vi "AlliGator Update Loaded Dataset Info.vi"(4 "Image Loading Options":T1={"Pixel Well Capacity"=0, "Pile-up Correction"=FALSE, "Gate Step"=0, "Image Smoothing Options"={"Use Image Smoothing"=FALSE, "Kernel Type"=enum."Bilinear", "Bin"=1, "Algorithm"=enum."Rapid"}, "Gates to Skip"={"Start"=0, "End"=0}, "File Background Subtraction"=FALSE, "Background File Path"=path "", "Image Binning Options"={"Use Image Binning"=FALSE, "X Bin"=1, "Y Bin"=1}, "# Gates"=0, "Gates to Keep"={"First"=0, "Last"=0}, "Define Gates to"=FALSE, "Hot Pixel Removal"={"Remove Screamers"=FALSE, "Delta"=0.0, "Equalize Histogram"=FALSE, "Percentile"=0.0, "Hot Pixel Mask Image"=path "", "Use Hot Pixel Mask"=FALSE}, "Dataset Scaling Factor"=0.0, "Image Pre-processing Steps"=[]} {"Hot Pixel Removal"."Percentile" min=0 max=100; "Image Binning Options"."Y Bin" min=1; "Image Binning Options"."X Bin" min=1; "Image Smoothing Options"."Bin" min=1}, 6 "Background File?":bool, 7 "Pile-up Correction":bool, 8 "error in (no error)":errorcluster, 9 "After Loading Dataset Information":T10, 10 "# Gates":i32, 11 "Pixel Well Capacity":u32) -> (0 "Error Out":errorcluster)   [LabVIEW 2021, in "AlliGator Files.lvlib"]
doc: "Updates Settings and Internal Variables after loading a new dataset."
uses:
  AlliGator Files.lvlib
  AlliGator After Loading Dataset Information.ctl
  AlliGator Image Loading Options.ctl
  AlliGator Image Smoothing Options.ctl
  Arrays/Kernel Type.ctl
  Arrays/Smoothing Algorithm.ctl
  AlliGator Gates to Skip.ctl
  AlliGator Image Binning Options.ctl
  AlliGator Gates to Keep.ctl
  SwissSPAD/SwissSPAD Live_Image Display Options.ctl
  AlliGator Image Pre-processing Step.ctl
  AlliGator Variables List.ctl
  AlliGator Settings List.ctl
  AlliGator Refnums List.ctl
  AlliGator Globals, Variables & Constants.lvlib
  AlliGator Settings.lvlib
  AlliGator GUI.lvlib
  Arrays/Arrays.lvlib
  AlliGator Decay Analysis.lvlib
  AlliGator Source Image.lvlib
  SwissSPAD/SwissSPAD Live.lvlib
panel:
  # "see the AlliGator License on the block diagram (Ctrl+E or Window:Show Block Diagram)"
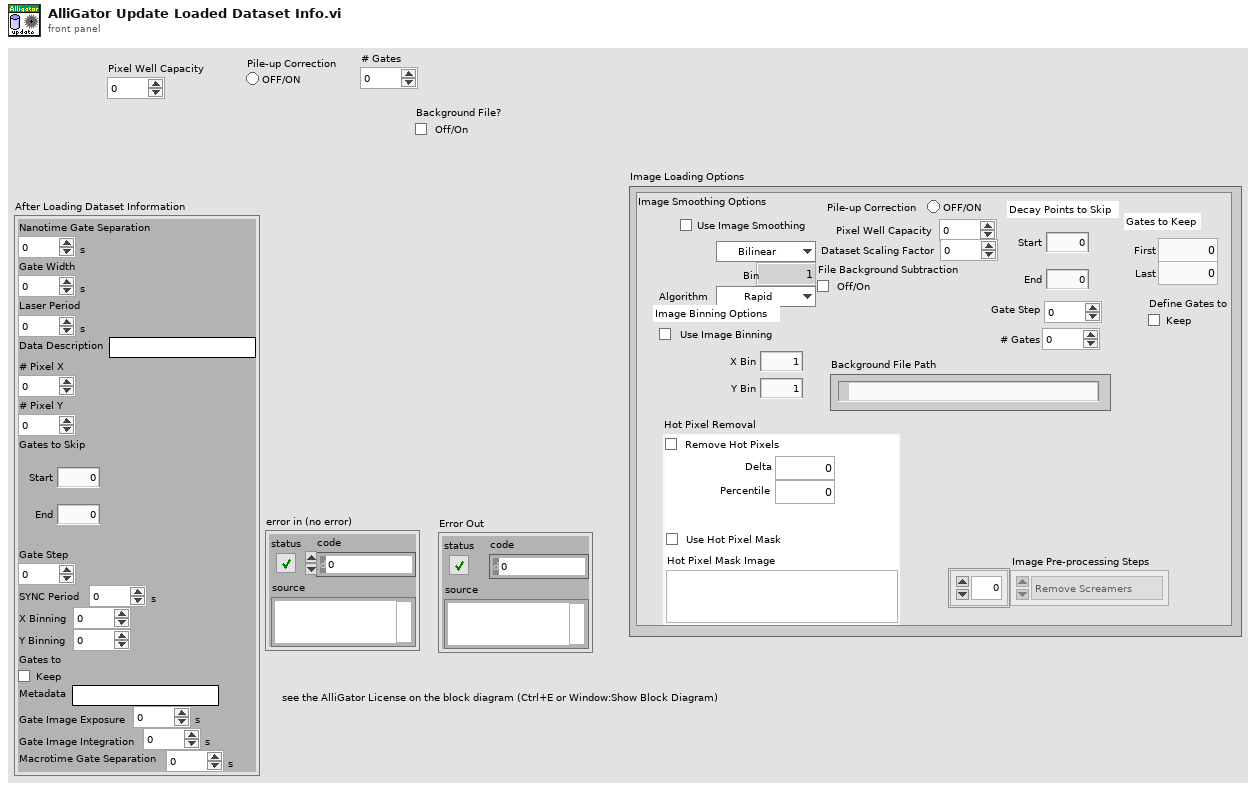
[diagram p1: front panel]
types:
  T1 = typedef "AlliGator Source Image.lvlib/AlliGator Image Loading Options.ctl" = cluster{"Pixel Well Capacity":u32, "Pile-up Correction":bool, "Gate Step":i32, "Image Smoothing Options":T2, "Gates to Skip":T5, "File Background Subtraction":bool, "Background File Path":path, "Image Binning Options":T6, "# Gates":u32, "Gates to Keep":T7, "Define Gates to":bool, "Hot Pixel Removal":T8, "Dataset Scaling Factor":dbl, "Image Pre-processing Steps":T9[]}
  T2 = typedef "AlliGator Settings.lvlib/AlliGator Image Smoothing Options.ctl" = cluster{"Use Image Smoothing":bool, "Kernel Type":T3, "Bin":i32, "Algorithm":T4}
  T3 = typedef "Arrays.lvlib/Kernel Type.ctl" = enum16{"Uniform", "Bilinear", "Gaussian"}
  T4 = typedef "Arrays.lvlib/Smoothing Algorithm.ctl" = enum16{"Rapid", "Thorough"}
  T5 = typedef "AlliGator Decay Analysis.lvlib/AlliGator Gates to Skip.ctl" = cluster{"Start":u32, "End":u32}
  T6 = typedef "AlliGator Source Image.lvlib/AlliGator Image Binning Options.ctl" = cluster{"Use Image Binning":bool, "X Bin":i32, "Y Bin":i32}
  T7 = typedef "AlliGator Settings.lvlib/AlliGator Gates to Keep.ctl" = cluster{"First":u32, "Last":u32}
  T8 = typedef "SwissSPAD Live.lvlib/SwissSPAD Live_Image Display Options.ctl" = cluster{"Remove Screamers":bool, "Delta":sgl, "Equalize Histogram":bool, "Percentile":sgl, "Hot Pixel Mask Image":path, "Use Hot Pixel Mask":bool}
  T9 = typedef "AlliGator Files.lvlib/AlliGator Image Pre-processing Step.ctl" = enum16{"Remove Screamers", "Pile-up Correction", "Binning", "Smoothing", "Rescaling", "Dead Left Column Correction"}
  T10 = typedef "AlliGator Files.lvlib/AlliGator After Loading Dataset Information.ctl" = cluster{"Nanotime Gate Separation":dbl[unit], "Gate Width":dbl[unit], "Laser Period":dbl[unit], "Data Description":string, "# Pixel X":i32, "# Pixel Y":i32, "Gates to Use":cluster{"Start":u32, "End":u32}, "Gate Step":i32, "SYNC Period":dbl[unit], "X Binning":i32, "Y Binning":i32, "Gates to":bool, "Metadata":string, "Gate Image Exposure":dbl[unit], "Gate Image Integration":dbl[unit], "Macrotime Gate Separation":dbl[unit]}
  T11 = typedef "AlliGator Globals, Variables & Constants.lvlib/AlliGator Variables List.ctl" = enum16{"---- GUI ----", "Initialization Status", "State Indicators Refnum", "Original AlliGator Menu Items", "Current Action Loop State", "Script in progress", "Playback", "Loop Playback", "Search ROI Used", "Search ROI", "Decay Graph Max Legend Size", "Intensity Graph Max Legend Size", "Decay Statistics Graph Max Legend Size", "Phasor Graph Max Legend Size", "Phasor Ratio Graph Max Legend Size", "Lifetime Graph Max Legend Size", "---- Files ----", "Export Dataset Frames as Individual Files", "Show Batch Export Help Balloons", "Frames in Dataset", "ptu File Frame Start Indices", "Current Frame in Dataset", "Current Frame Timestamp", "------ Python Plugins ------", "Python Plugins Information", "Python Session", "Valid Python Session?", "---- Source Image ----", "Dataset Loaded", "Dataset Metadata", "Dataset Channel", "Dataset Data Description", "Background Dataset Metadata", "Background Dataset Channel", "Background Dataset Data Description", "Background File Subtraction", "Background File Path", "Background File Pile-up Correction", "Background File Pixel Well Capacity", "Background File Scaling Factor", "Source Image ROIs", "Current Source Image ROI", "Source Image ROI Event Refnum", "X_Source Image Display Range", "X_Source Image Palette Information", "Source Image Palette List", "Source Image Scale", "Current Dataset Load Settings", "Source Image:ROI Overlay Color", "---- Image Profile Window ----", "Image Profile:Overlay ROI in Source Image", "Image Profile Window Event Refnum", "Image Profile:IntensityType", "Image Profile:Intensity Average Type", "Image Profile:Intensity-weighted SDV", "Image Profile:Box Profile Type", "Image Profile Window Open", "Image Profile:Plotted Fit Parameter", "X_Type of Displayed Image", "X_Time Gate Slider", "Dataset Path", "Source Image Overlay to Erase", "Is Displayed Image Accumulated", "White Light Image Modified", "Mask Image Modified", "Macrotime Gate Separation", "------ Phasor Graph -------", "Phasor Graph:Show Line", "---- Phasor Plot ---", "Phasor Plot Parameters Changed", "FLI Dataset Modified since last Phasor Plot Calculation", "Phasor Harmonics Data", "Selected Phasor Harmonics", "Phasor Harmonic Manager Event Refnum", "Phasor Plot ROIs", "Current Phasor Plot ROI", "Phasor Plot ROI Event Refnum", "Phasor Plot Image Reference Points", "Phasor Plot Computed", "Phasor Plot Palette Information", "Phasor Plot Palette List", "Phasor Ratio Palette Information", "Phasor Ratio Palette List", "Phasor Image Scale", "Phasor Plot Image Overlay to Erase", "Phasor Plot Image Elements to Update", "Current Phasor Plot Calculation Parameters", "Current Phasor Calibration Options", "Reset Cumulated Phasor Plot", "Phasor Ratio Reference 1", "Phasor Ratio Lifetime Reference 1", "Phasor Ratio Reference 1 Frequency", "Phasor Ratio Reference 2", "Phasor Ratio Lifetime Reference 2", "Phasor Ratio Reference 2 Frequency", "---- Decay Analysis ----", "Number of Selected Decays to Fit", "LS Fit Results", "LAR Fit Results", "BS Fit Results", "Last Decay Max - Min", "Best Fit Parameters", "Best Fit Parameter Names", "Actual Size X", "Actual Size Y", "Binning X", "Binning Y", "Actual # Gates", "Dataset Number", "Gates to...", "Gates Skipped", "Gates to keep", "Gate Step", "Gate Separation", "Reversed Gates", "Pile-up Correction", "Pixel Well Capacity", "Background Subtracted", "Background Subtraction Method", "Background Definition Range", "Background File (deprecated)", "Number of Dataset Accumulated", "Array of Accumulated Dataset Paths", "Do Averaged Datasets", "Destination File Path", "Process Plot Target", "Use 1/D as Phasor Frequency", "---- Decay Fit Parameter Map -----", "Decay Fit Parameter Map Palette Information", "Decay Fit Parameter Map Palette List", "Local Decay Graph Window Event Refnum", "------- Local Decay Window ---------", "Use normalized IRF for convolution", "----- Miscellaneous ----", "Skippable Dialog Windows Status"}
  T12 = typedef "AlliGator Settings.lvlib/AlliGator Settings List.ctl" = enum16{"GUI:Visible Settings Tab", "GUI:Last Run Version", "Source Image:Use Image Histogram for Contrast", "Source Image:Low Count Pixels Rejection Options", "Source Image:High Count Pixels Rejection Options", "Source Image:Use Image Brightness", "Source Image:Blend Overlay with Image Background", "Source Image:Use Fixed ROI Diameter", "Source Image:ROI Diameter", "Source Image:ROI Center Color", "Source Image:Peak Threshold", "Source Image:Intensity Threshold", "Source Image:Image Binning Options", "Source Image:Image Smoothing Options", "Source Image:Image Histogram Active", "Source Image:Invert Binary Mask", "Source Image:Hot Pixel Removal", "Source Image:Overlay Analyzed ROI Center", "Source Image:Auto-Adjust Contrast", "Source Image:Histogram Lower Percentile", "Source Image:Histogram Upper Percentile", "Source Image:Save Source Image", "Source Image:Scale Bar Options", "Source Image:Image Resolution (Pixel Size)", "Source Image:Flatfield Correction", "Source Image:Show Dead Left Columns Correction", "Source Image:Dead Left Columns Correction", "Source Image:Image Pre-Processing Operations Order", "Data Information:Gate Width", "Data Information:Nanotime Gate Separation", "Data Information:Macrotime Gate Separation", "Data Information:Gate Step", "Data Information:# Gates", "Data Information:Gate Image Exposure", "Data Information:Gate Image Integration", "Data Information:Gates to Skip", "Data Information:Gates to Keep", "Data Information:Define Gates to", "Data Information:Channel Name", "Data Information:Available Channel Names", "Data Information:Channel Arithmetic", "Data Information:Background File Subtraction", "Data Information:Background File", "Data Information:Background Scaling Factor", "Data Information:Background Pile-up Correction", "Data Information:Background Pixel Well Capacity", "Data Information:Laser Period", "Data Information:SYNC Period", "Data Information:Pile-up Correction", "Data Information:Pixel Well Capacity", "Data Information:Dataset Scaling Factor", "Fluorescence Decay_Decay Pre-Processing:Reverse Gates", "Fluorescence Decay_Decay Pre-Processing:Verbose Decay Pre-Processing", "Fluorescence Decay_Decay Pre-Processing:Use Decay Pre-Processing", "Fluorescence Decay_Decay Pre-Processing:Background Subtraction", "Fluorescence Decay_Decay Pre-Processing:Background Definition Range", "Fluorescence Decay_Decay Pre-Processing:Baseline Subtraction Method", "Fluorescence Decay_Decay Pre-Processing:Decay Pre-Processing Operations Order", "Fluorescence Decay_Decay Pre-Processing:Smoothing Parameter", "Fluorescence Decay_Decay Pre-Processing:Shift Decay", "Fluorescence Decay_Decay Pre-Processing:Decay Shift Parameters", "Fluorescence Decay_Decay Pre-Processing:Fold Decay", "Fluorescence Decay_Decay Pre-Processing:# Folds", "Fluorescence Decay_Decay Pre-Processing:1-Normalize Decay", "Fluorescence Decay_Decay Pre-Processing:[0-1]-Normalize Decay", "Fluorescence Decay_Decay Pre-Processing:Smoothen Decay", "Fluorescence Decay_Decay Pre-Processing:Extrapolate Decay", "Fluorescence Decay_Decay Pre-Processing:Use Periodicity", "Fluorescence Decay_Decay Pre-Processing:Use Cursors", "Fluorescence Decay_Decay Pre-Processing:Tail Fraction", "Fluorescence Decay_Decay Pre-Processing:Head Fraction", "Fluorescence Decay_Decay Pre-Processing:Additional Points", "Fluorescence Decay_Decay Pre-Processing:Straighten Decay", "Fluorescence Decay_Decay Pre-Processing:Constant Background", "Fluorescence Decay_Decay Pre-Processing:Pixel-Normalize Decay", "Fluorescence Decay_Advanced Analysis:Extract IRF instead of Decay", "Fluorescence Decay_Advanced Analysis:IRF Extraction Options", "Fluorescence Decay_Advanced Analysis:IRF Optimization Options", "Fluorescence Decay_Advanced Analysis:Square Pulse Options", "Fluorescence Decay_Advanced Analysis:IRF Order", "Fluorescence Decay_Advanced Analysis:IRF Time Constants", "Fluorescence Decay_Advanced Analysis:Wavelet Analysis Options", "Fluorescence Decay_Advanced Analysis:Average Lifetime Options", "Fluorescence Decay_Fit Options:Fit Options", "Fluorescence Decay_Fit Options:Use Legacy Fitting Approach", "Fluorescence Decay_Fit Options:Use Data Information Laser Period", "Fluorescence Decay_Fit Parameters:Displayed Fit Parameters", "Fluorescence Decay_Fit Parameters:Fit Parameter Constraints", "Fluorescence Decay_Fit Parameters:Export Tabulated Results", "Fluorescence Decay_Fit Parameters:MLE Baseline Offset Type", "Fluorescence Decay_Fit Parameters:MLE Baseline Offset", "Fluorescence Decay_Fit Parameters:Guess Parameter Names", "Fluorescence Decay_Fit Parameters:Guess Parameter Values", "Fluorescence Decay_Fit Parameters:Guess Parameters Options", "Fluorescence Decay_Styles:Show Last Decay Only", "Fluorescence Decay_Styles:Decay Graph Color Array", "Fluorescence Decay:Decay Graph Active", "Fluorescence Decay Statistics:Min Peak Value", "Fluorescence Decay Statistics:Reject Low Decay Peak Pixels", "Fluorescence Decay Statistics:Reject High Decay Peak Pixels", "Fluorescence Decay Statistics:Max Peak Value", "Time Traces:Use File Timestamp", "Time Traces:Time Step", "Time Traces:Use Intensity Correction File", "Time Traces:Intensity Correction File", "Phasor Plot:Phasor Plot Smoothing Options", "Phasor Plot:Phasor Plot Size", "Phasor Plot:Phasor Plot Graphics Options", "Phasor Plot:Cumulative Phasor Plot", "Phasor Plot:Use Phasor Brightness", "Phasor Plot:Blend Overlay with Phasor Background", "Phasor Plot:Save Phasor Plot", "Phasor Plot:Show References", "Phasor Plot:Phasor Ratio Decay Range", "Phasor Plot:Exponential Fading", "Phasor Plot:Phasor Ratio Reference Colors", "Phasor Plot:Reference Radius", "Phasor Plot:Show Color Map Vertices", "Phasor Plot:Phasor Plot Active", "Phasor Plot:Phasor Ratio Color Map Type", "Phasor Plot:Phasor Ratio Color Map", "Phasor Plot:Phasor Ratio Display Range", "Phasor Plot:Selected Image ROI(s)", "Phasor Plot:All Image ROIs", "Phasor Plot:Selected Phasor Plot ROI(s)", "Phasor Plot:All Phasor Plot ROIs", "Phasor Plot:Phasor Ratio Color-Coded Quantity", "Phasor Plot:Store Phasor Harmonics", "Phasor Plot:Draw Reference Segment", "Phasor Plot:User-Defined Quantity", "Phasor Graph:Phasor Frequency", "Phasor Graph:Phasor Ratio Type", "Phasor Graph:Pixel-level Phasor Computation", "Phasor Graph:Save Phasor Graph", "Phasor Graph:Phasor Graph Active", "Phasor Graph:Phasor SDV Options", "Phasor Calibration:Use Backup Calibration if needed", "Phasor Graph:Define Shortest Lifetime as", "Phasor Calibration:Backup Calibration Type", "Phasor Calibration:Calibration Type", "Phasor Calibration:Calibration Lifetime", "Phasor Calibration:Calibration Map Algorithm", "Single-Exponential Phasor Locus (SEPL):Gate Parameters", "Single-Exponential Phasor Locus (SEPL):User-defined Gate", "Single-Exponential Phasor Locus (SEPL):User-defined IRF", "Single-Exponential Phasor Locus (SEPL):Phasor Parameters", "Single-Exponential Phasor Locus (SEPL):Decay & IRF Parameters", "Single-Exponential Phasor Locus (SEPL):Display Parameters", "Lifetime Analysis:Decay Analysis Parameters", "Lifetime Analysis:Lifetime Map Active", "Plugins:Python Settings", "Miscellaneous:Verbose Mode", "Miscellaneous:Beep after Script", "Miscellaneous:Saved Image File Format", "Miscellaneous:Exported Gate Image Settings", "Miscellaneous:Include Loading in Timing", "Miscellaneous:Verbose Settings Mode", "Miscellaneous:Histogram Options", "Miscellaneous:Beep on Error", "Miscellaneous:# Logical Processors Used", "Miscellaneous:ROI Description Max Characters", "Miscellaneous:Verbose Error Mode", "Miscellaneous:Transparent Mask Color"}
  T13 = typedef "AlliGator Globals, Variables & Constants.lvlib/AlliGator Refnums List.ctl" = enum16{"---------- AlliGator Controls ----------", "AlliGator Tab Control Refnum", "---------- AlliGator Indicators ----------", "Source Image Display Refnum", "Phasor Plot Display Refnum", "Decay Fit Parameter Map Refnum", "---------- AlliGator VIs ----------", "AlliGator Settings Refnum", "AlliGator Launcher Refnum"}
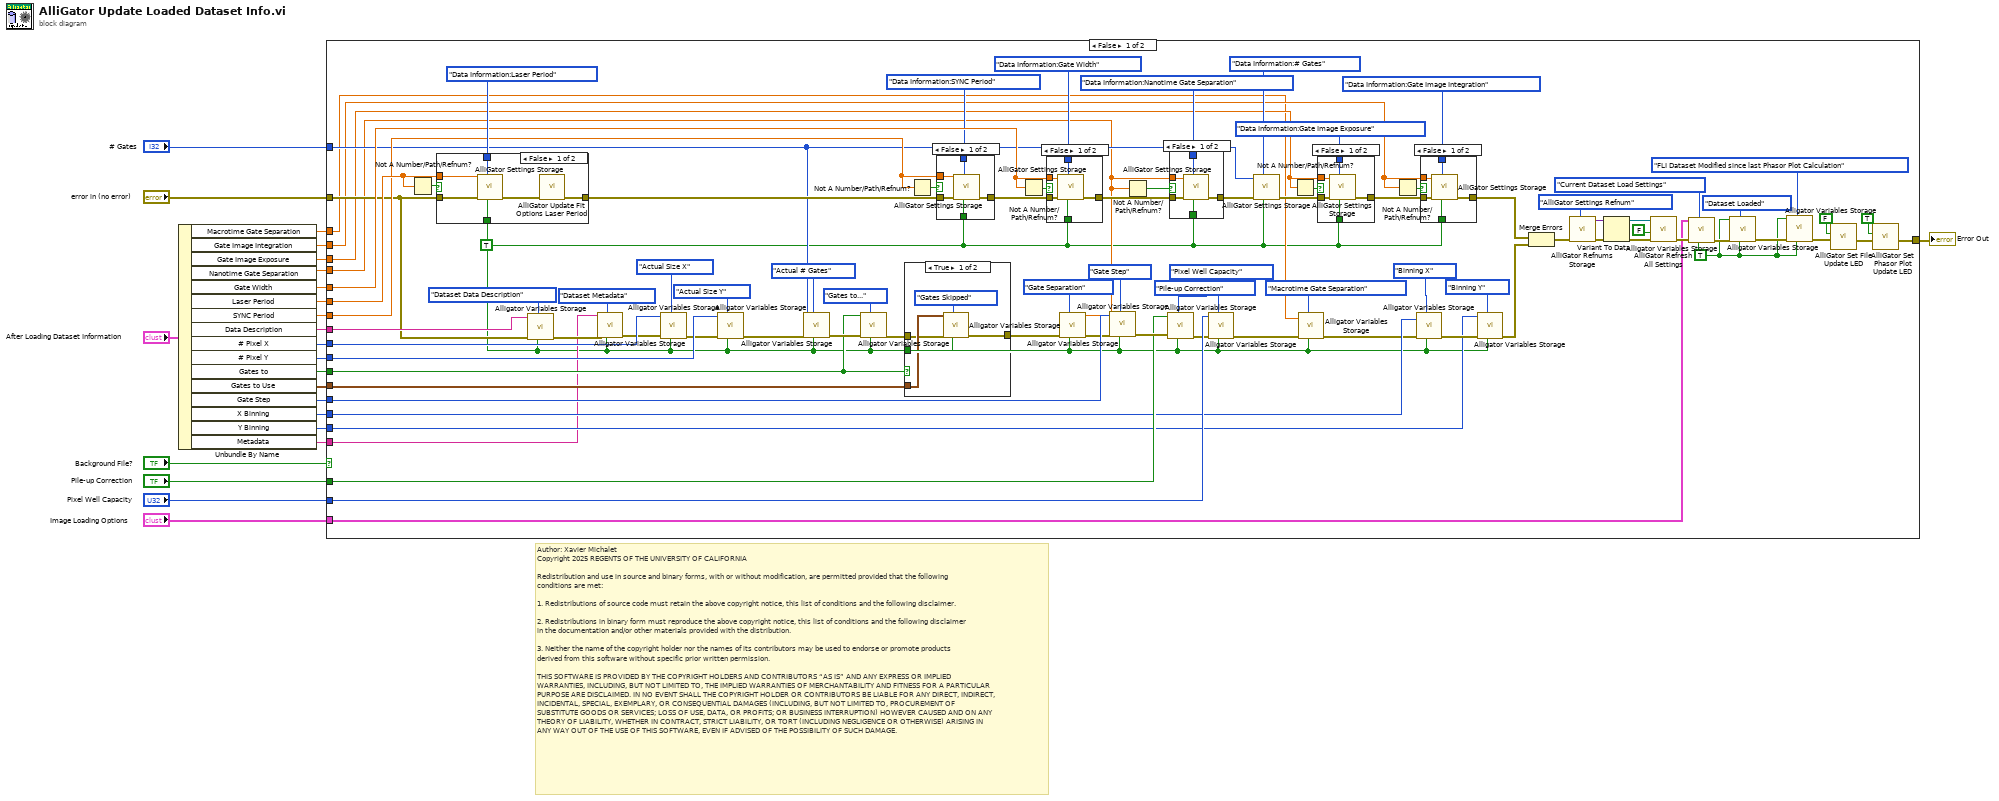
[diagram p0: block diagram]
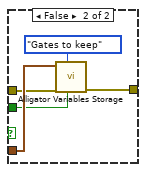
[diagram p6: hidden frame]
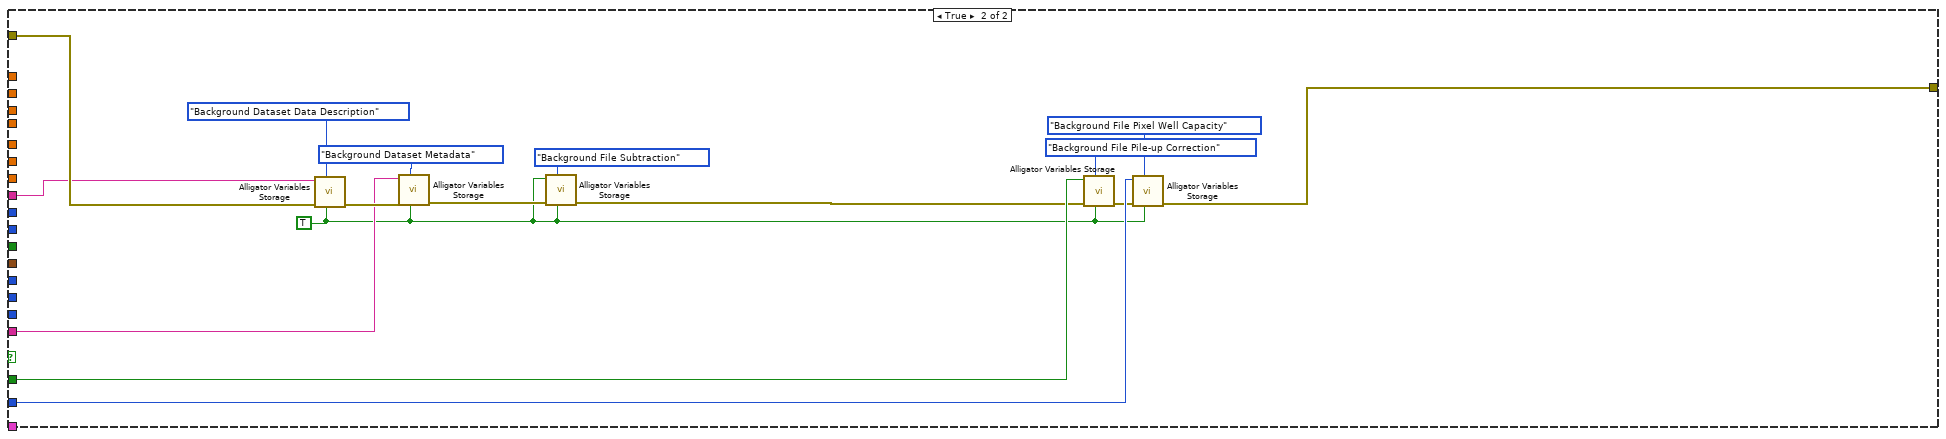
[diagram p9: hidden frame]
diagram:
  # "Author: Xavier Michalet\nCopyright 2025 REGENTS OF THE UNIVERSITY OF CALIFORNIA\n\nRedistribution and use in source and binary forms, with or without modification, are permitted provided that the following conditions are met:\n\n1. Redistributions of source code must retain the above copyright notice, this list of conditions and the following disclaimer.\n\n2. Redistributions in binary form must reproduce the above copyright notice, this list of conditions and the following disclaimer in the documentation and/or other materials provided with the distribution.\n\n3. Neither the name of the copyright holder nor the names of its contributors may be used to endorse or promote products derived from this software without specific prior written permission.\n\nTHIS SOFTWARE IS PROVIDED BY THE COPYRIGHT HOLDERS AND CONTRIBUTORS “AS IS” AND ANY EXPRESS OR IMPLIED WARRANTIES, INCLUDING, BUT NOT LIMITED TO, THE IMPLIED WARRANTIES OF MERCHANTABILITY AND FITNESS FOR A PARTICULAR PURPOSE ARE DISCLAIMED. IN NO EVENT SHALL THE COPYRIGHT HOLDER OR CONTRIBUTORS BE LIABLE FOR ANY DIRECT, INDIRECT, INCIDENTAL, SPECIAL, EXEMPLARY, OR CONSEQUENTIAL DAMAGES (INCLUDING, BUT NOT LIMITED TO, PROCUREMENT OF SUBSTITUTE GOODS OR SERVICES; LOSS OF USE, DATA, OR PROFITS; OR BUSINESS INTERRUPTION) HOWEVER CAUSED AND ON ANY THEORY OF LIABILITY, WHETHER IN CONTRACT, STRICT LIABILITY, OR TORT (INCLUDING NEGLIGENCE OR OTHERWISE) ARISING IN ANY WAY OUT OF THE USE OF THIS SOFTWARE, EVEN IF ADVISED OF THE POSSIBILITY OF SUCH DAMAGE."
  n1 = Unbundle By Name("After Loading Dataset Information") -> ("Macrotime Gate Separation"=w1:dbl[unit], "Gate Image Integration"=w2:dbl[unit], "Gate Image Exposure"=w3:dbl[unit], "Nanotime Gate Separation"=w8:dbl[unit], "Gate Width"=w17:dbl[unit], "Laser Period"=w18:dbl[unit], "SYNC Period"=w15:dbl[unit], "Data Description"=w10:string, "# Pixel X"=w22:i32, "# Pixel Y"=w23:i32, "Gates to"=w11:bool, "Gates to Use"=w24:cluster{"Start":u32, "End":u32}, "Gate Step"=w14:i32, "X Binning"=w13:i32, "Y Binning"=w12:i32, "Metadata"=w4:string)
  n2 = case shown="False" "Background File?" {
    tunnel: w24 -> [w112 _]
    tunnel: w23 -> [w111 _]
    tunnel: w22 -> [w110 _]
    tunnel: "Pile-up Correction" -> [w106 w175]
    tunnel: "Pixel Well Capacity" -> [w105 w174]
    tunnel: w18 -> [w95 _]
    tunnel: w17 -> [w93 _]
    tunnel: "# Gates" -> [w40 _]
    tunnel: w15 -> [w85 _]
    tunnel: w14 -> [w81 _]
    tunnel: w13 -> [w76 _]
    tunnel: w12 -> [w75 _]
    tunnel: w11 -> [w64 _]
    tunnel: w10 -> [w63 w167]
    tunnel: "error in (no error)" -> [w61 w168]
    tunnel: w8 -> [w31 _]
    tunnel: [w53 w173] -> w6
    tunnel: "Image Loading Options" -> [w48 _]
    tunnel: w4 -> [w44 w169]
    tunnel: w3 -> [w33 _]
    tunnel: w2 -> [w32 _]
    tunnel: w1 -> [w27 _]
    frame False {
      w49 = TRUE ("Get(F)/Set")
      w25 = TRUE ("Get(F)/Set")
      n3 = Not A Number/Path/Refnum?(number/path/refnum=w95) -> (NaN/Path/Refnum?=w94:bool)
      n4 = case shown="False" w94 {
        tunnel: w25 -> [w158 _]
        tunnel: [w154 w159] -> w88
        tunnel: AlliGator_Settings_List."Data Information:Laser Period" ("AlliGator Settings List") -> [w157 _]
        tunnel: w95 -> [w153 _]
        tunnel: w61 -> [w156 w159]
        frame False {
          n5 = call "AlliGator Settings Storage.vi"("Get(F)/Set"=w158, "AlliGator Settings List"=w157, "Error In"=w156, "Variant Data in"=w153) -> ("Error Out"=w155:errorcluster)  [unwired: 6 in, 1 out]
          n6 = call "AlliGator Update Fit Options Laser Period.vi"("error in (no error)"=w155) -> ("error out"=w154:errorcluster)  [unwired: 10 in]
        }
        frame True {
        }
      }
      n7 = call "Alligator Variables Storage.vi"("Get(F)/Set"=w25, "AlliGator Variable"=AlliGator_Variables_List."Dataset Data Description" ("Alligator Variable"), "Error In"=w61, "Data in"=w63) -> ("Error Out"=w47:errorcluster)  [unwired: 5 in, 2 out]
      n8 = call "Alligator Variables Storage.vi"("Get(F)/Set"=w25, "AlliGator Variable"=AlliGator_Variables_List."Dataset Metadata" ("Alligator Variable"), "Error In"=w47, "Data in"=w44) -> ("Error Out"=w46:errorcluster)  [unwired: 5 in, 2 out]
      n9 = call "Alligator Variables Storage.vi"("Get(F)/Set"=w25, "AlliGator Variable"=AlliGator_Variables_List."Actual Size X" ("Alligator Variable"), "Error In"=w46, "Data in"=w110) -> ("Error Out"=w101:errorcluster)  [unwired: 5 in, 2 out]
      n10 = call "Alligator Variables Storage.vi"("Get(F)/Set"=w25, "AlliGator Variable"=AlliGator_Variables_List."Actual Size Y" ("Alligator Variable"), "Error In"=w101, "Data in"=w111) -> ("Error Out"=w103:errorcluster)  [unwired: 5 in, 2 out]
      n11 = call "Alligator Variables Storage.vi"("Get(F)/Set"=w25, "AlliGator Variable"=AlliGator_Variables_List."Actual # Gates" ("Alligator Variable"), "Error In"=w103, "Data in"=w40) -> ("Error Out"=w67:errorcluster)  [unwired: 5 in, 2 out]
      n12 = call "Alligator Variables Storage.vi"("Get(F)/Set"=w25, "AlliGator Variable"=AlliGator_Variables_List."Gates to..." ("Alligator Variable"), "Error In"=w67, "Data in"=w64) -> ("Error Out"=w66:errorcluster)  [unwired: 5 in, 2 out]
      n13 = case shown="True" w64 {
        tunnel: w112 -> [w141 w146]
        tunnel: [w139 w144] -> w83
        tunnel: w66 -> [w138 w143]
        tunnel: w25 -> [w137 w142]
        frame True {
          n14 = call "Alligator Variables Storage.vi"("Get(F)/Set"=w137, "AlliGator Variable"=AlliGator_Variables_List."Gates Skipped" ("Alligator Variable"), "Error In"=w138, "Data in"=w141) -> ("Error Out"=w139:errorcluster)  [unwired: 5 in, 2 out]
        }
        frame False {
          n15 = call "Alligator Variables Storage.vi"("Get(F)/Set"=w142, "AlliGator Variable"=AlliGator_Variables_List."Gates to keep" ("Alligator Variable"), "Error In"=w143, "Data in"=w146) -> ("Error Out"=w144:errorcluster)  [unwired: 5 in, 2 out]
        }
      }
      n16 = Not A Number/Path/Refnum?(number/path/refnum=w85) -> (NaN/Path/Refnum?=w86:bool)
      n17 = case shown="False" w86 {
        tunnel: w25 -> [w151 _]
        tunnel: [w150 w152] -> w87
        tunnel: AlliGator_Settings_List."Data Information:SYNC Period" ("AlliGator Settings List") -> [w149 _]
        tunnel: w85 -> [w148 _]
        tunnel: w88 -> [w147 w152]
        frame False {
          n18 = call "AlliGator Settings Storage.vi"("Get(F)/Set"=w151, "AlliGator Settings List"=w149, "Error In"=w147, "Variant Data in"=w148) -> ("Error Out"=w150:errorcluster)  [unwired: 6 in, 1 out]
        }
        frame True {
        }
      }
      n19 = Not A Number/Path/Refnum?(number/path/refnum=w93) -> (NaN/Path/Refnum?=w92:bool)
      n20 = case shown="False" w92 {
        tunnel: w25 -> [w135 _]
        tunnel: [w134 w136] -> w107
        tunnel: AlliGator_Settings_List."Data Information:Gate Width" ("AlliGator Settings List") -> [w133 _]
        tunnel: w87 -> [w132 w136]
        tunnel: w93 -> [w131 _]
        frame False {
          n21 = call "AlliGator Settings Storage.vi"("Get(F)/Set"=w135, "AlliGator Settings List"=w133, "Error In"=w132, "Variant Data in"=w131) -> ("Error Out"=w134:errorcluster)  [unwired: 6 in, 1 out]
        }
        frame True {
        }
      }
      n22 = call "Alligator Variables Storage.vi"("Get(F)/Set"=w25, "AlliGator Variable"=AlliGator_Variables_List."Gate Separation" ("Alligator Variable"), "Error In"=w83, "Data in"=w31) -> ("Error Out"=w68:errorcluster)  [unwired: 5 in, 2 out]
      n23 = call "Alligator Variables Storage.vi"("Get(F)/Set"=w25, "AlliGator Variable"=AlliGator_Variables_List."Gate Step" ("Alligator Variable"), "Error In"=w68, "Data in"=w81) -> ("Error Out"=w108:errorcluster)  [unwired: 5 in, 2 out]
      n24 = Not A Number/Path/Refnum?(number/path/refnum=w31) -> (NaN/Path/Refnum?=w91:bool)
      n25 = call "Alligator Variables Storage.vi"("Get(F)/Set"=w25, "AlliGator Variable"=AlliGator_Variables_List."Pile-up Correction" ("Alligator Variable"), "Error In"=w108, "Data in"=w106) -> ("Error Out"=w41:errorcluster)  [unwired: 5 in, 2 out]
      n26 = case shown="False" w91 {
        tunnel: [w129 w130] -> w89
        tunnel: w25 -> [w128 _]
        tunnel: w107 -> [w127 w130]
        tunnel: AlliGator_Settings_List."Data Information:Nanotime Gate Separation" ("AlliGator Settings List") -> [w126 _]
        tunnel: w31 -> [w125 _]
        frame False {
          n27 = call "AlliGator Settings Storage.vi"("Get(F)/Set"=w128, "AlliGator Settings List"=w126, "Error In"=w127, "Variant Data in"=w125) -> ("Error Out"=w129:errorcluster)  [unwired: 6 in, 1 out]
        }
        frame True {
        }
      }
      n28 = call "Alligator Variables Storage.vi"("Get(F)/Set"=w25, "AlliGator Variable"=AlliGator_Variables_List."Pixel Well Capacity" ("Alligator Variable"), "Error In"=w41, "Data in"=w105) -> ("Error Out"=w29:errorcluster)  [unwired: 5 in, 2 out]
      n29 = call "AlliGator Settings Storage.vi"("Get(F)/Set"=w25, "AlliGator Settings List"=AlliGator_Settings_List."Data Information:# Gates", "Error In"=w89, "Variant Data in"=w40) -> ("Error Out"=w37:errorcluster)  [unwired: 6 in, 1 out]
      n30 = Not A Number/Path/Refnum?(number/path/refnum=w33) -> (NaN/Path/Refnum?=w39:bool)
      n31 = call "Alligator Variables Storage.vi"("Get(F)/Set"=w25, "AlliGator Variable"=AlliGator_Variables_List."Macrotime Gate Separation" ("Alligator Variable"), "Error In"=w29, "Data in"=w27) -> ("Error Out"=w28:errorcluster)  [unwired: 5 in, 2 out]
      n32 = case shown="False" w39 {
        tunnel: w25 -> [w123 _]
        tunnel: [w122 w124] -> w36
        tunnel: AlliGator_Settings_List."Data Information:Gate Image Exposure" ("AlliGator Settings List") -> [w121 _]
        tunnel: w37 -> [w120 w124]
        tunnel: w33 -> [w119 _]
        frame False {
          n33 = call "AlliGator Settings Storage.vi"("Get(F)/Set"=w123, "AlliGator Settings List"=w121, "Error In"=w120, "Variant Data in"=w119) -> ("Error Out"=w122:errorcluster)  [unwired: 6 in, 1 out]
        }
        frame True {
        }
      }
      n34 = Not A Number/Path/Refnum?(number/path/refnum=w32) -> (NaN/Path/Refnum?=w38:bool)
      n35 = call "Alligator Variables Storage.vi"("Get(F)/Set"=w25, "AlliGator Variable"=AlliGator_Variables_List."Binning X" ("Alligator Variable"), "Error In"=w28, "Data in"=w76) -> ("Error Out"=w80:errorcluster)  [unwired: 5 in, 2 out]
      n36 = case shown="False" w38 {
        tunnel: w25 -> [w117 _]
        tunnel: [w116 w118] -> w30
        tunnel: AlliGator_Settings_List."Data Information:Gate Image Integration" ("AlliGator Settings List") -> [w115 _]
        tunnel: w36 -> [w114 w118]
        tunnel: w32 -> [w113 _]
        frame False {
          n37 = call "AlliGator Settings Storage.vi"("Get(F)/Set"=w117, "AlliGator Settings List"=w115, "Error In"=w114, "Variant Data in"=w113) -> ("Error Out"=w116:errorcluster)  [unwired: 6 in, 1 out]
        }
        frame True {
        }
      }
      n38 = call "Alligator Variables Storage.vi"("Get(F)/Set"=w25, "AlliGator Variable"=AlliGator_Variables_List."Binning Y" ("Alligator Variable"), "Error In"=w80, "Data in"=w75) -> ("Error Out"=w79:errorcluster)  [unwired: 5 in, 2 out]
      n39 = Merge Errors(w30, w79) -> (w71:errorcluster)
      n40 = call "AlliGator Refnums Storage.vi"("AlliGator Refnum List"=AlliGator_Refnums_List."AlliGator Settings Refnum", "Error In"=w71) -> ("Error Out"=w73:errorcluster, "Data out"=w72:variant)  [unwired: 8 in]
      n41 = Variant To Data(error in=w73, Variant=w72) -> (data=w69:refnum<vi>, error out=w70:errorcluster)  [unwired: 1 in]
      n42 = call "AlliGator Refresh All Settings.vi"("Error In"=w70, "Verbose (T)"=FALSE, "VI Refnum in"=w69) -> ("Error Out"=w55:errorcluster)  [unwired: 8 in]
      n43 = call "Alligator Variables Storage.vi"("Get(F)/Set"=w49, "AlliGator Variable"=AlliGator_Variables_List."Current Dataset Load Settings" ("Alligator Variable"), "Error In"=w55, "Data in"=w48) -> ("Error Out"=w59:errorcluster)  [unwired: 5 in, 2 out]
      n44 = call "Alligator Variables Storage.vi"("Get(F)/Set"=w49, "AlliGator Variable"=AlliGator_Variables_List."Dataset Loaded" ("Alligator Variable"), "Error In"=w59, "Data in"=w49) -> ("Error Out"=w52:errorcluster)  [unwired: 5 in, 2 out]
      n45 = call "Alligator Variables Storage.vi"("Get(F)/Set"=w49, "AlliGator Variable"=AlliGator_Variables_List."FLI Dataset Modified since last Phasor Plot Calculation" ("Alligator Variable"), "Error In"=w52, "Data in"=w49) -> ("Error Out"=w51:errorcluster)  [unwired: 5 in, 2 out]
      n46 = call "AlliGator Set File Update LED.vi"("error in (no error)"=w51, "Off/On"=FALSE) -> ("error out"=w57:errorcluster)  [unwired: 9 in]
      n47 = call "AlliGator Set Phasor Plot Update LED.vi"("error in (no error)"=w57, "Off/On"=TRUE) -> ("error out"=w53:errorcluster)  [unwired: 9 in]
    }
    frame True {
      w160 = TRUE ("Get(F)/Set")
      n48 = call "Alligator Variables Storage.vi"("Get(F)/Set"=w160, "AlliGator Variable"=AlliGator_Variables_List."Background Dataset Data Description" ("Alligator Variable"), "Error In"=w168, "Data in"=w167) -> ("Error Out"=w171:errorcluster)  [unwired: 5 in, 2 out]
      n49 = call "Alligator Variables Storage.vi"("Get(F)/Set"=w160, "AlliGator Variable"=AlliGator_Variables_List."Background Dataset Metadata" ("Alligator Variable"), "Error In"=w171, "Data in"=w169) -> ("Error Out"=w163:errorcluster)  [unwired: 5 in, 2 out]
      n50 = call "Alligator Variables Storage.vi"("Get(F)/Set"=w160, "AlliGator Variable"=AlliGator_Variables_List."Background File Subtraction" ("Alligator Variable"), "Error In"=w163, "Data in"=w160) -> ("Error Out"=w162:errorcluster)  [unwired: 5 in, 2 out]
      n51 = call "Alligator Variables Storage.vi"("Get(F)/Set"=w160, "AlliGator Variable"=AlliGator_Variables_List."Background File Pile-up Correction" ("Alligator Variable"), "Error In"=w162, "Data in"=w175) -> ("Error Out"=w164:errorcluster)  [unwired: 5 in, 2 out]
      n52 = call "Alligator Variables Storage.vi"("Get(F)/Set"=w160, "AlliGator Variable"=AlliGator_Variables_List."Background File Pixel Well Capacity" ("Alligator Variable"), "Error In"=w164, "Data in"=w174) -> ("Error Out"=w173:errorcluster)  [unwired: 5 in, 2 out]
    }
  }
  "Error Out" <- w6
